vi "Handle_Space_Mouse_Input.vi"(6 "SpaceMouse_Buttons":T1, 7 "SpaceMouse_FilteredInput in":T2, 8 "error in (no error)":errorcluster, 9 "Attitude_Increase_Speed":dbl=2.0 format="%#_13g", 10 "old desired Attitude":T3, 11 "Attitude Control on":bool) -> (0 "error out":errorcluster, 2 "New desired Attitude":T3, 3 "SpaceMouse or Controller Output":T2)   [LabVIEW 2013]
uses:
  Controls/SpaceMouse_FilteredInput.ctl
  Controls/SpaceMouse_Buttons.ctl
  Controls/Steering Inputs.ctl
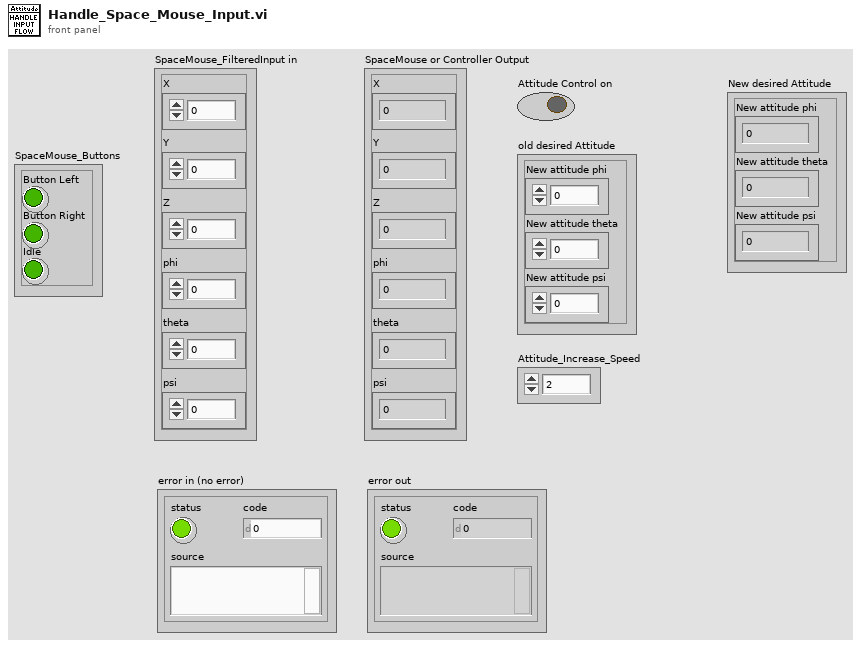
[diagram p1: front panel]
types:
  T1 = typedef "SpaceMouse_Buttons.ctl" = cluster{"Idle":bool, "Button Right":bool, "Button Left":bool}
  T2 = typedef "SpaceMouse_FilteredInput.ctl" = cluster{"X":dbl, "Y":dbl, "Z":dbl, "phi":dbl, "theta":dbl, "psi":dbl}
  T3 = cluster{"New attitude phi":dbl, "New attitude theta":dbl, "New attitude psi":dbl}
  T4 = typedef "Steering Inputs.ctl" = cluster{"X":dbl, "Y":dbl, "Z":dbl, "phi":dbl, "theta":dbl, "psi":dbl}
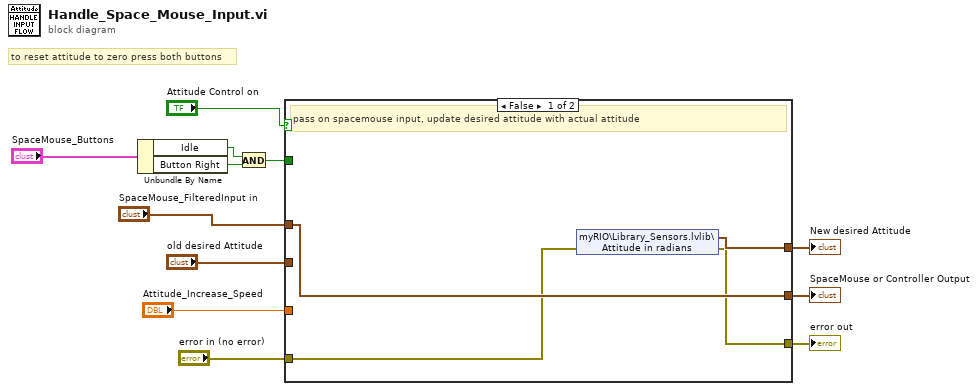
[diagram p0: block diagram]
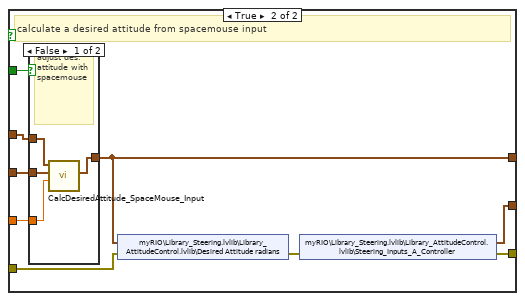
[diagram p2: hidden frame]
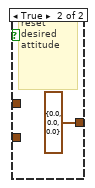
[diagram p3: hidden frame]
diagram:
  # "to reset attitude to zero press both buttons"
  n1 = Unbundle By Name("SpaceMouse_Buttons") -> ("Idle"=w3:bool, "Button Right"=w2:bool)
  n2 = And(x=w3, y=w2) -> (x .and. y?=w1:bool)
  n3 = case shown="False" "Attitude Control on" {
    tunnel: "SpaceMouse_FilteredInput in" -> [w16 w25]
    tunnel: [w16 w22] -> w8
    tunnel: "error in (no error)" -> [w14 w19]
    tunnel: [w15 w24] -> w11
    tunnel: [w13 w18] -> w10
    tunnel: "old desired Attitude" -> [_ w23]
    tunnel: "Attitude_Increase_Speed" -> [_ w20]
    tunnel: w1 -> [_ w17]
    frame False {
      # "pass on spacemouse input, update desired attitude with actual attitude"
      n4 = shared-variable "myRIO\\Library_Sensors.lvlib\\Attitude in radians"(error in=w14) -> (w15:cluster{"Roll":dbl, "Pitch":dbl, "Yaw":dbl}, error out=w13:errorcluster)
    }
    frame True {
      # "calculate a desired attitude from spacemouse input"
      n5 = case shown="False" w17 {
        tunnel: w25 -> [w29 _]
        tunnel: [w28 T3 {"New attitude phi"=0.0, "New attitude theta"=0.0, "New attitude psi"=0.0} ("New desired Attitude")] -> w24
        tunnel: w23 -> [w27 _]
        tunnel: w20 -> [w26 _]
        frame False {
          # "adjust des. attitude with spacemouse"
          n6 = call "CalcDesiredAttitude_SpaceMouse_Input.vi"("Attitude_Increase_Speed"=w26, "Old desired Attitude"=w27, "SpaceMouse_FilteredInput"=w29) -> ("New desired Attitude"=w28:T3)  [unwired: 8 in]
        }
        frame True {
          # "reset desired attitude"
        }
      }
      n7 = shared-variable "myRIO\\Library_Steering.lvlib\\Library_AttitudeControl.lvlib\\Desired Attitude radians"(w24, error in=w19) -> (error out=w21:errorcluster)
      n8 = shared-variable "myRIO\\Library_Steering.lvlib\\Library_AttitudeControl.lvlib\\Steering_Inputs_A_Controller"(error in=w21) -> (w22:T4, error out=w18:errorcluster)
    }
  }
  "New desired Attitude" <- w11
  "error out" <- w10
  "SpaceMouse or Controller Output" <- w8
